vi "Command - On-Demand (SubVI) - B.vi"(0 "ESP Config":T2={"COM Port Input"="COM8", "Manual Command"={"Device Type"="", "Instance"="", "Command"="", "Sub-Command"="", "Parameters (Seperate by :)"=""}, "Device Type"="e", "Instance"="a", "Use Manual Command"=TRUE, "Timeout [msec]"=1000, "Read/Write Wait [msec]"=25}, 5 "ESP Table Cluster Ref":refnum<vi>, 7 "Display Cluster Ref":refnum<vi>) -> (4 "ESP Output":T3={"Write Command"="ea:DU:1", "Read String"="\u0006\u0001ea:00.000:00.000:00.036:00.004:AEA8\u0004", "Read Bytes"=12, "Bytes at Port"=12, "Response"="ea:00.000:00.000:00.036:00.004:AEA8", "ACK"=TRUE, "EOT"=TRUE, "NAK"=FALSE, "Parameters"=["00.000", "00.000", "00.036", "00.004"]}, 8 "On-Demand Header":string[](array[string]), 10 "On-Demand Data":string[](array[string]), 15 "ON Demand":errorcluster={"status"=FALSE, "code"=1073676294, "source"="VISA Read in ESP-D Read-Write (SubVI).vi->IO Board Evaluate.vi"})   [LabVIEW 2011]
panel:
  out "data 2":i32[](array[numeric])
  out "data":T1(array[cluster])
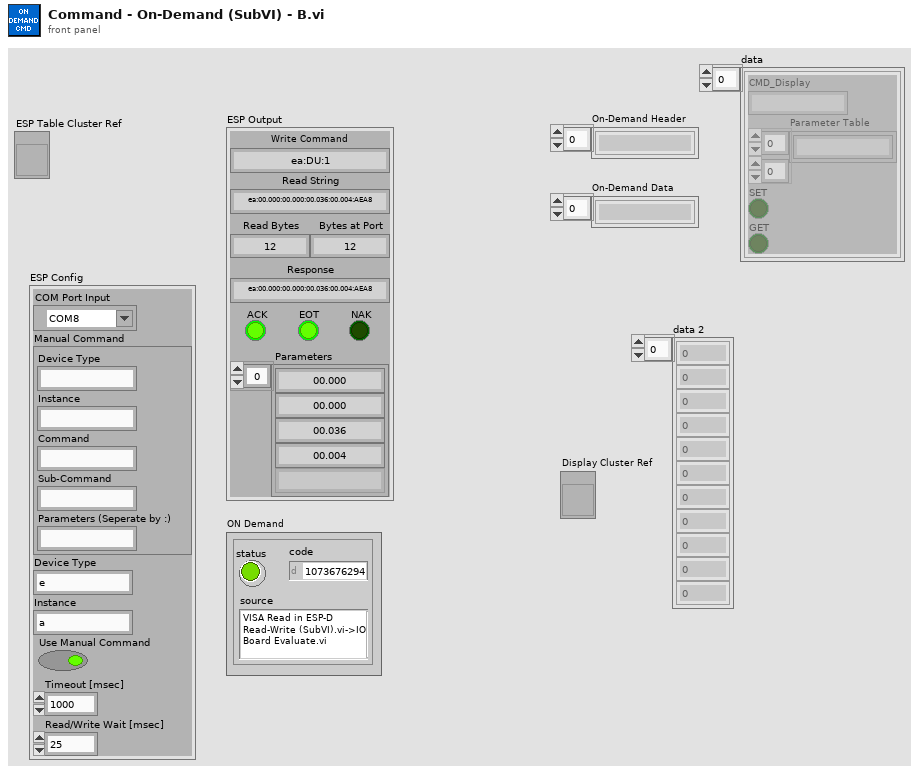
[diagram p1: front panel]
types:
  T1 = cluster{"CMD_Display":string, "Parameter Table":string[][], "SET":bool, "GET":bool}[]
  T2 = cluster{"COM Port Input":refnum<visa-resource-name>, "Manual Command":cluster{"Device Type":string, "Instance":string, "Command":string, "Sub-Command":string, "Parameters (Seperate by :)":string}, "Device Type":string, "Instance":string, "Use Manual Command":bool, "Timeout [msec]":u32, "Read/Write Wait [msec]":u32}
  T3 = cluster{"Write Command":string, "Read String":string, "Read Bytes":u32, "Bytes at Port":u32, "Response":string, "ACK":bool, "EOT":bool, "NAK":bool, "Parameters":string[]}
  T4 = cluster{"ON Demand Button":i32, "ON Demand Commands":i32, "Continuous Button":i32, "Continuous Commands":i32, "Error Button":i32, "Error Command":i32, "Status Button":i32, "Status Command":i32, "Digital Button":i32, "Digital Command":i32, "Save Table Button":i32, "Active Table":i32, "New Table Name":i32, "Table":i32}
  T5 = cluster{"Device Type":string, "Instance":string, "Command":string, "Sub-Command":string, "Parameters (Seperate by :)":string}
  T6 = cluster{"CMD_Display":string, "Parameter Table":string[][], "SET":bool, "GET":bool}
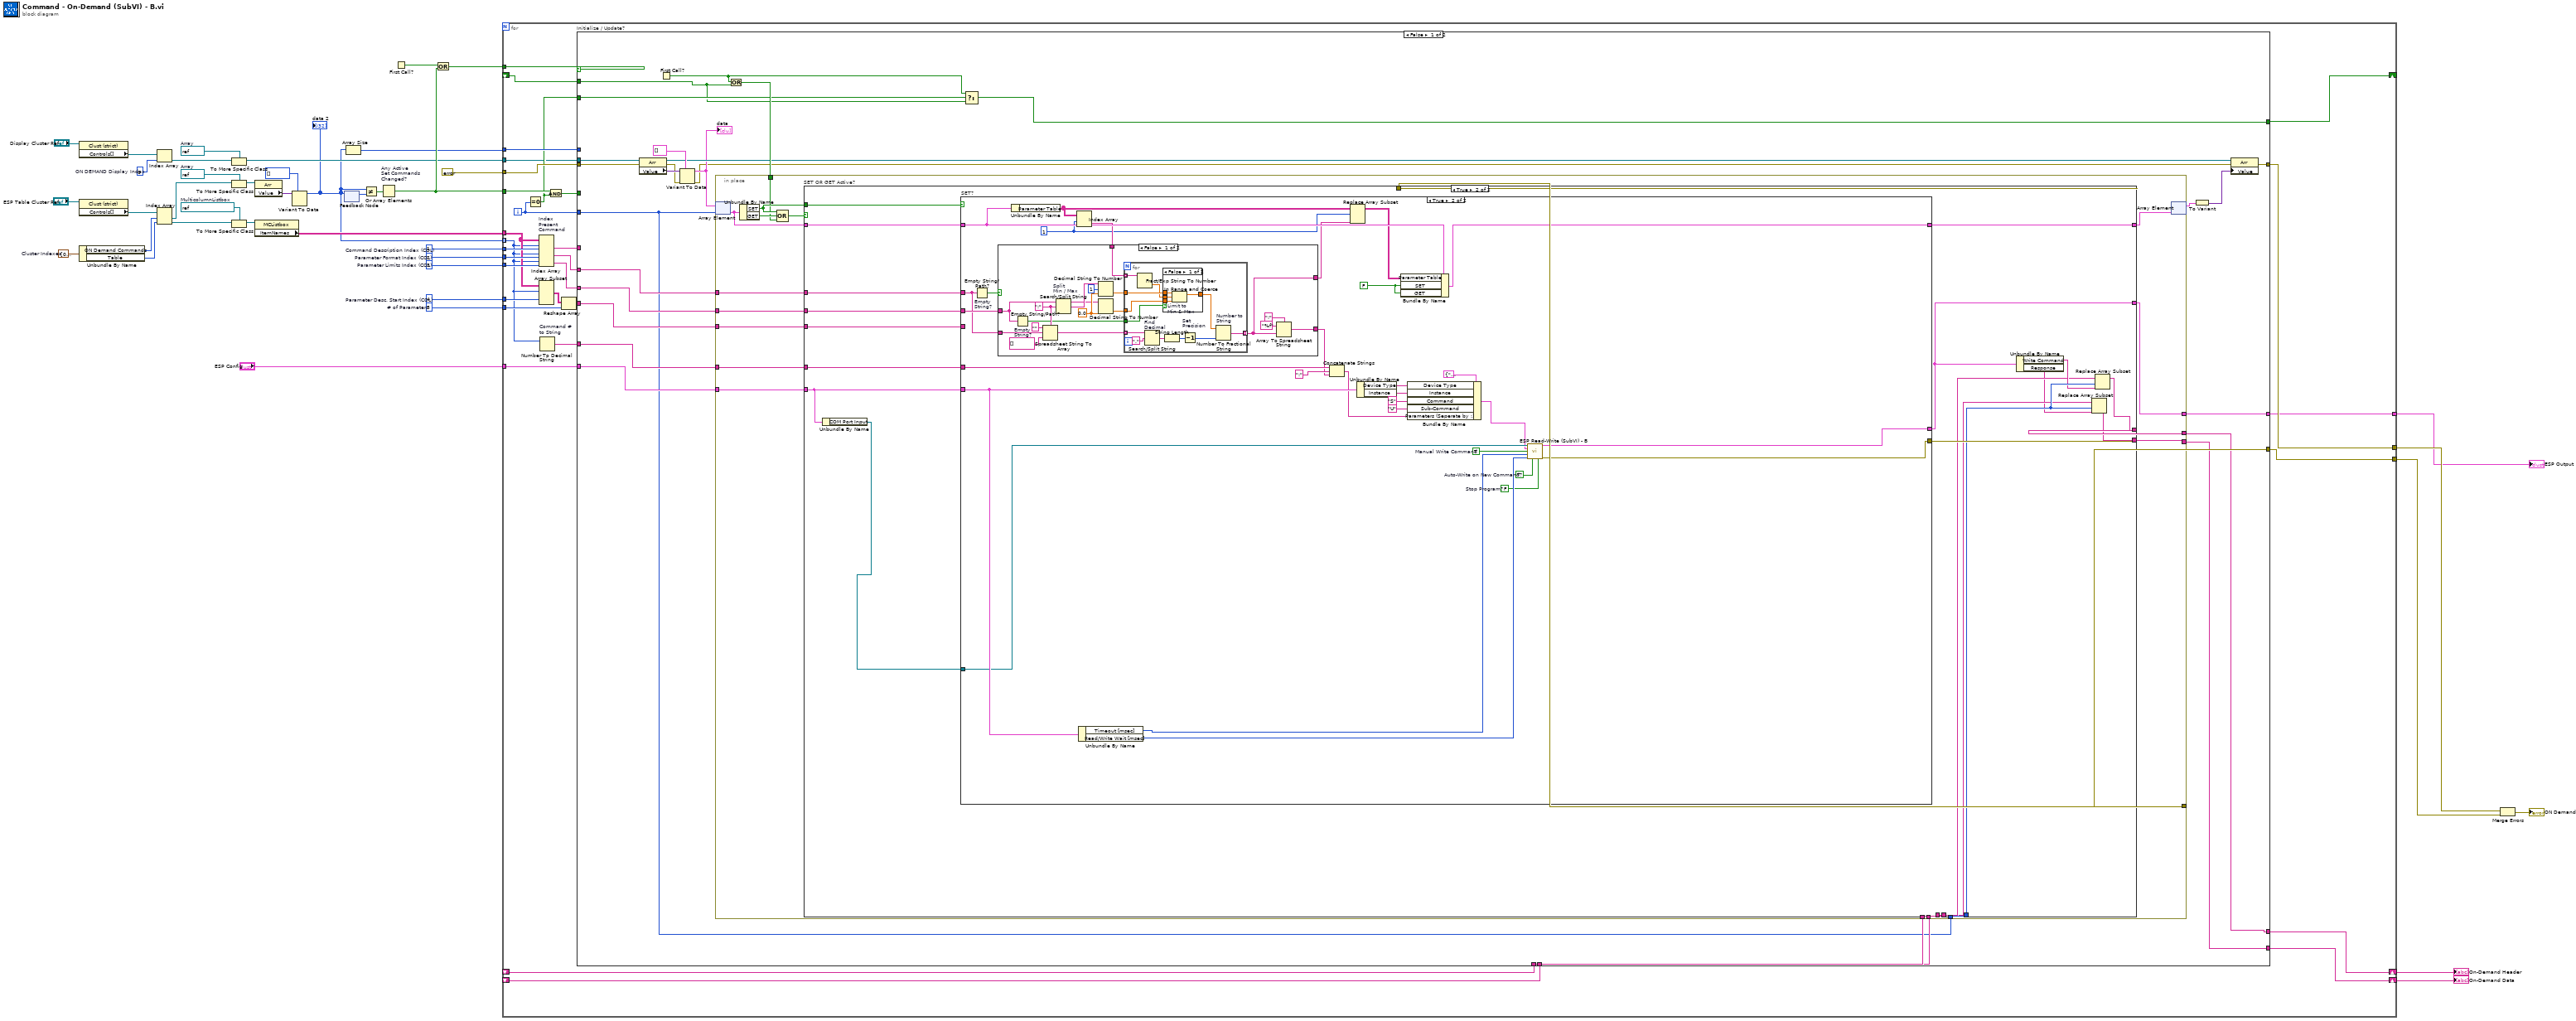
[diagram p0: block diagram]
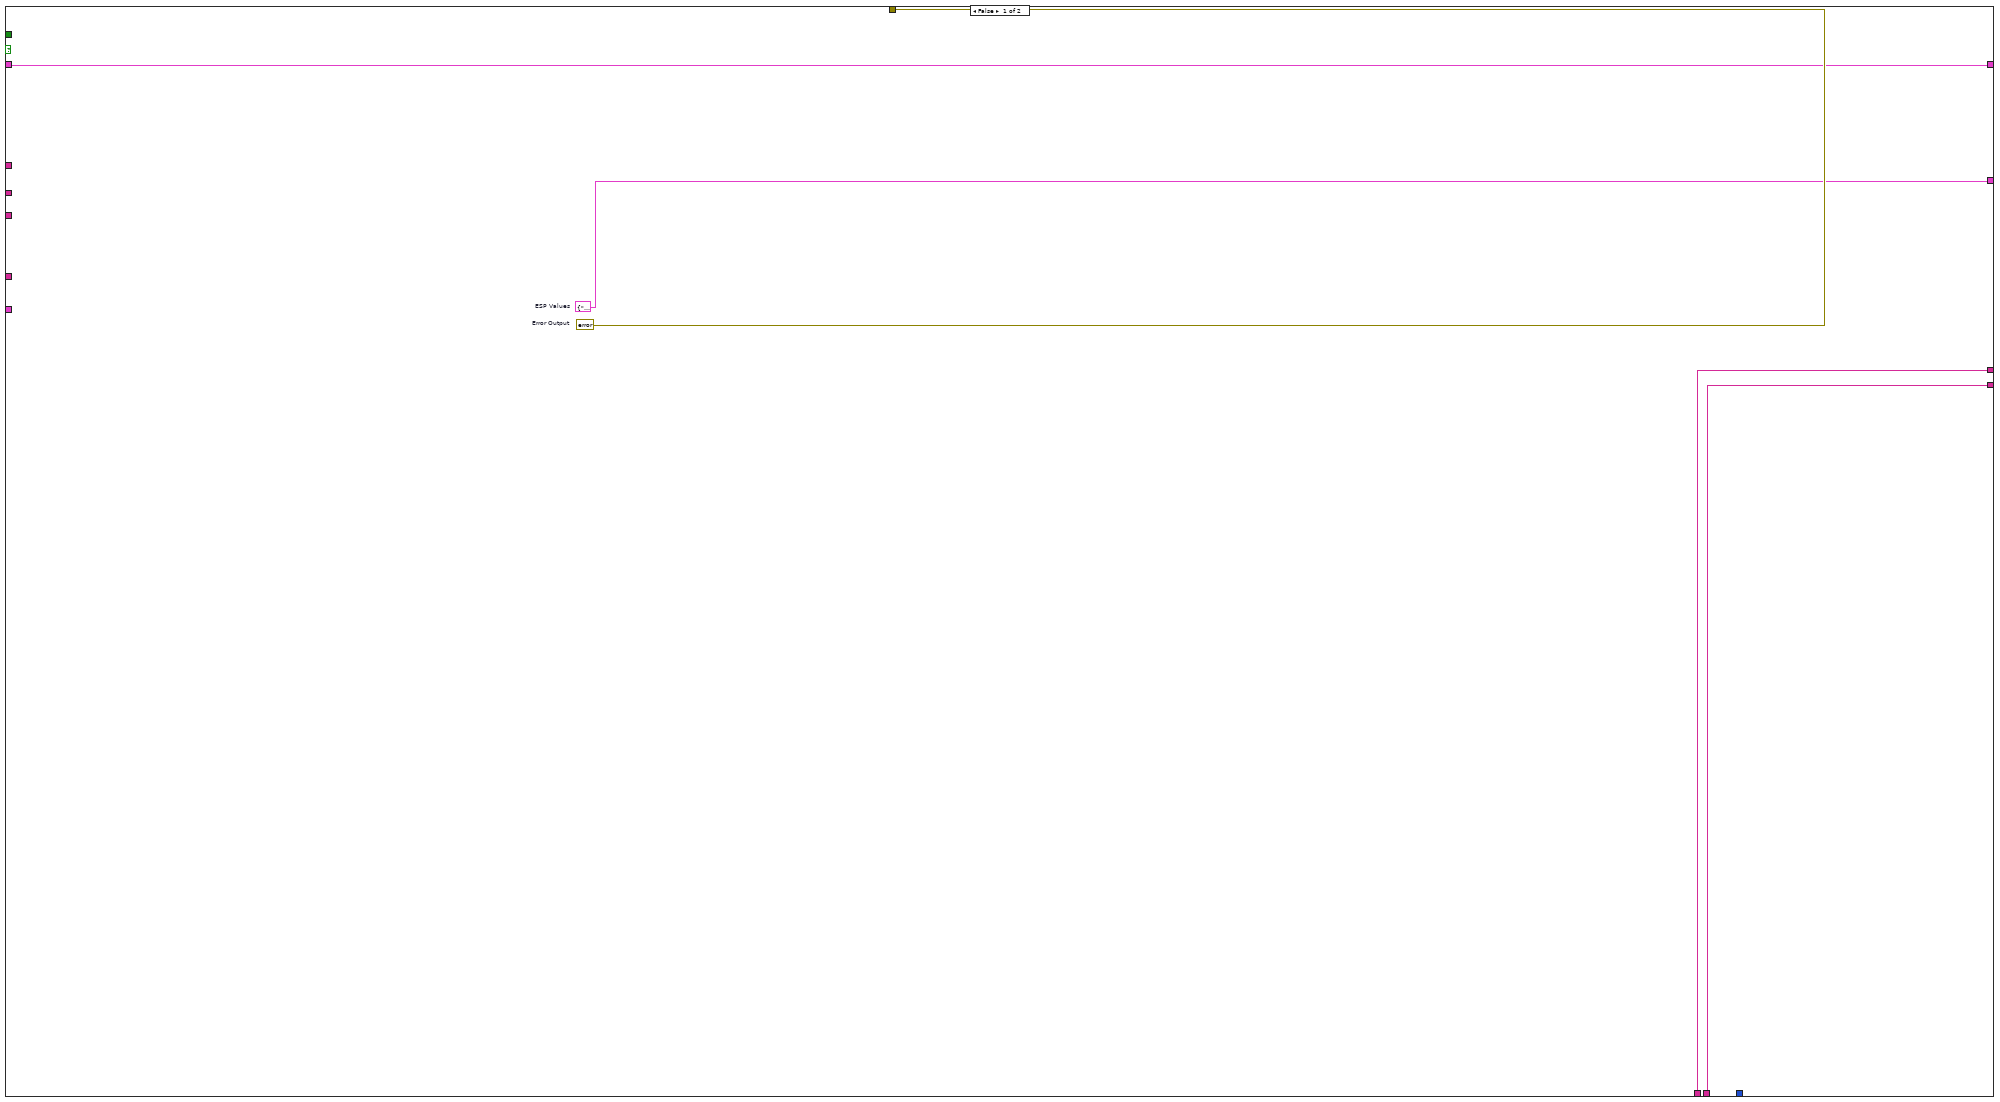
[diagram p2: hidden frame]
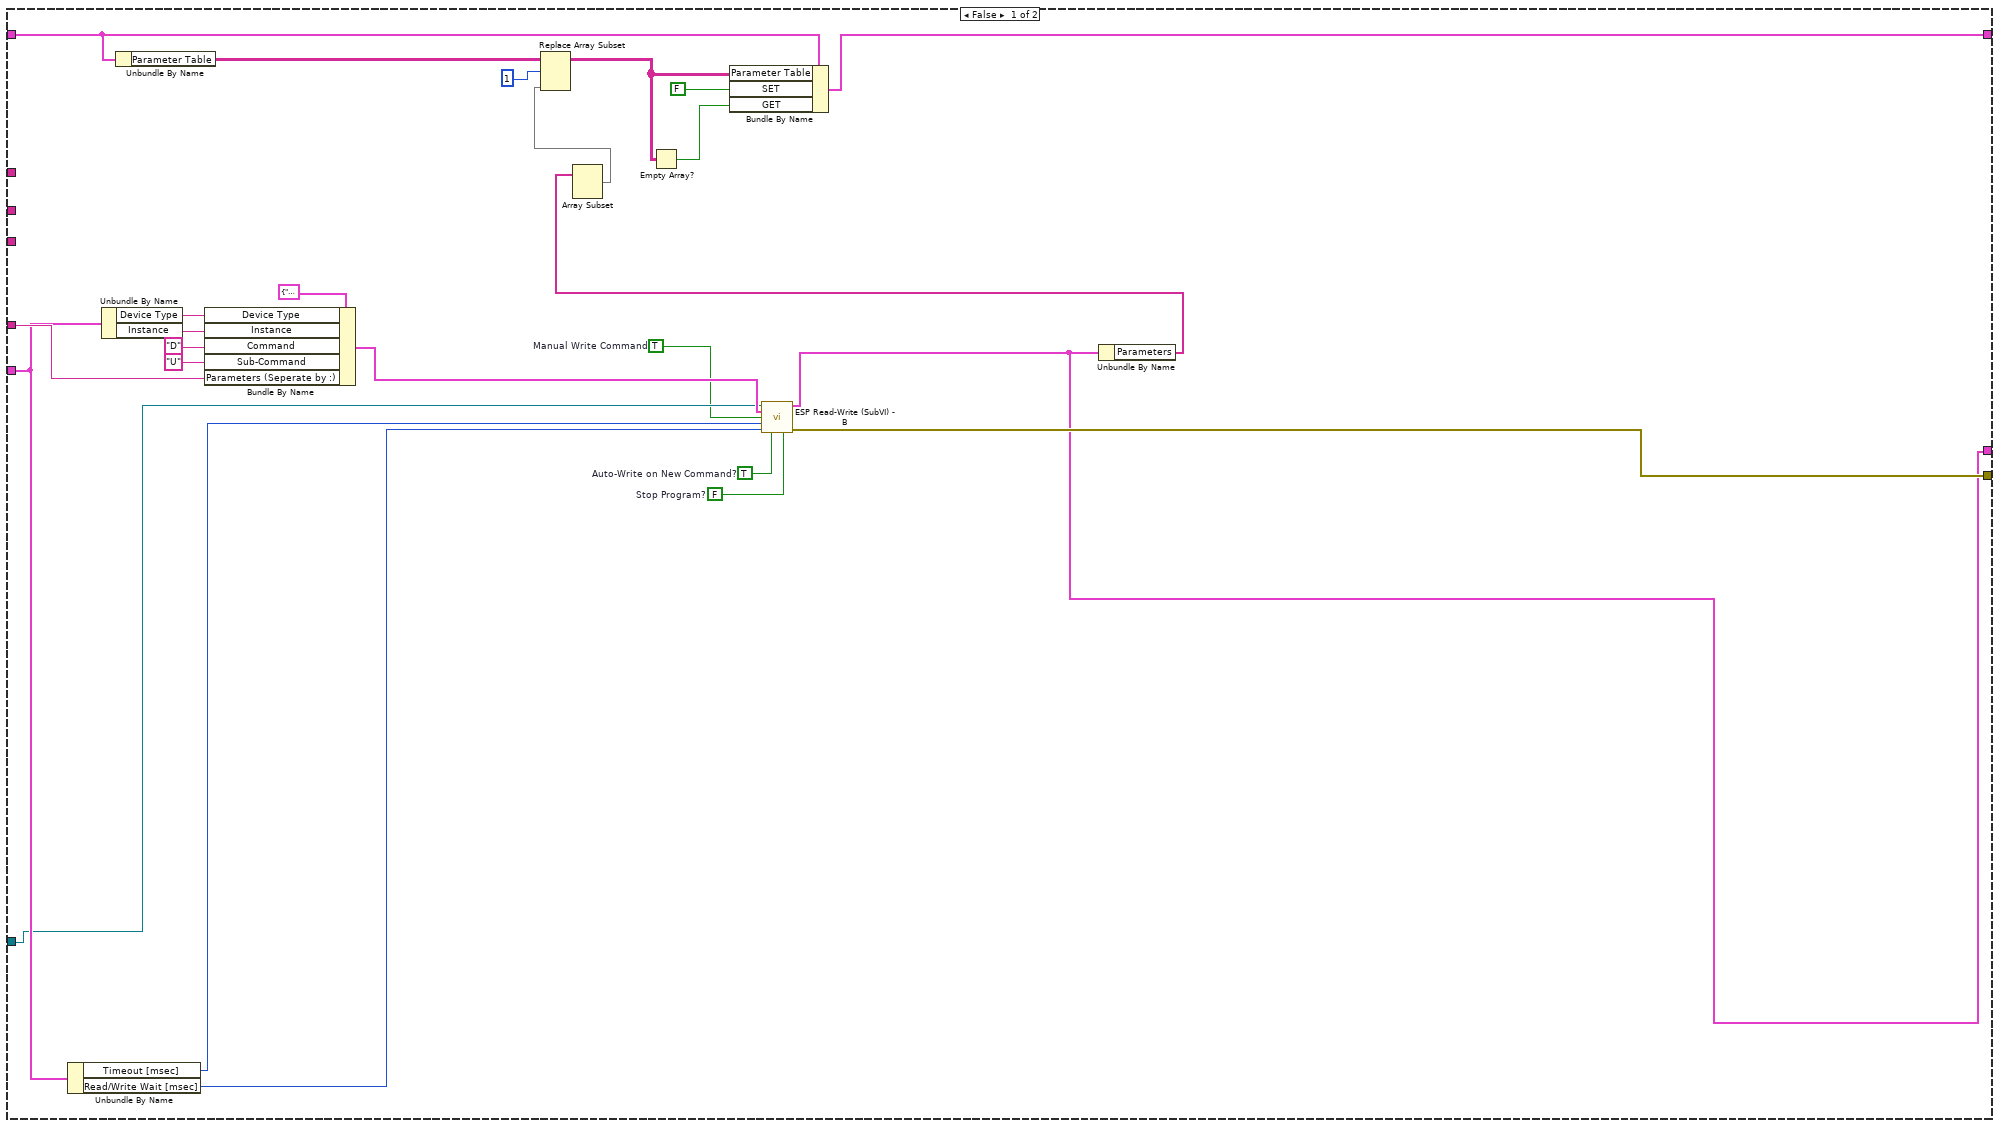
[diagram p3: hidden frame]
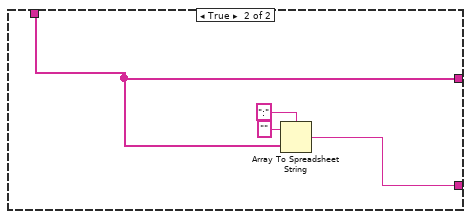
[diagram p5: hidden frame]
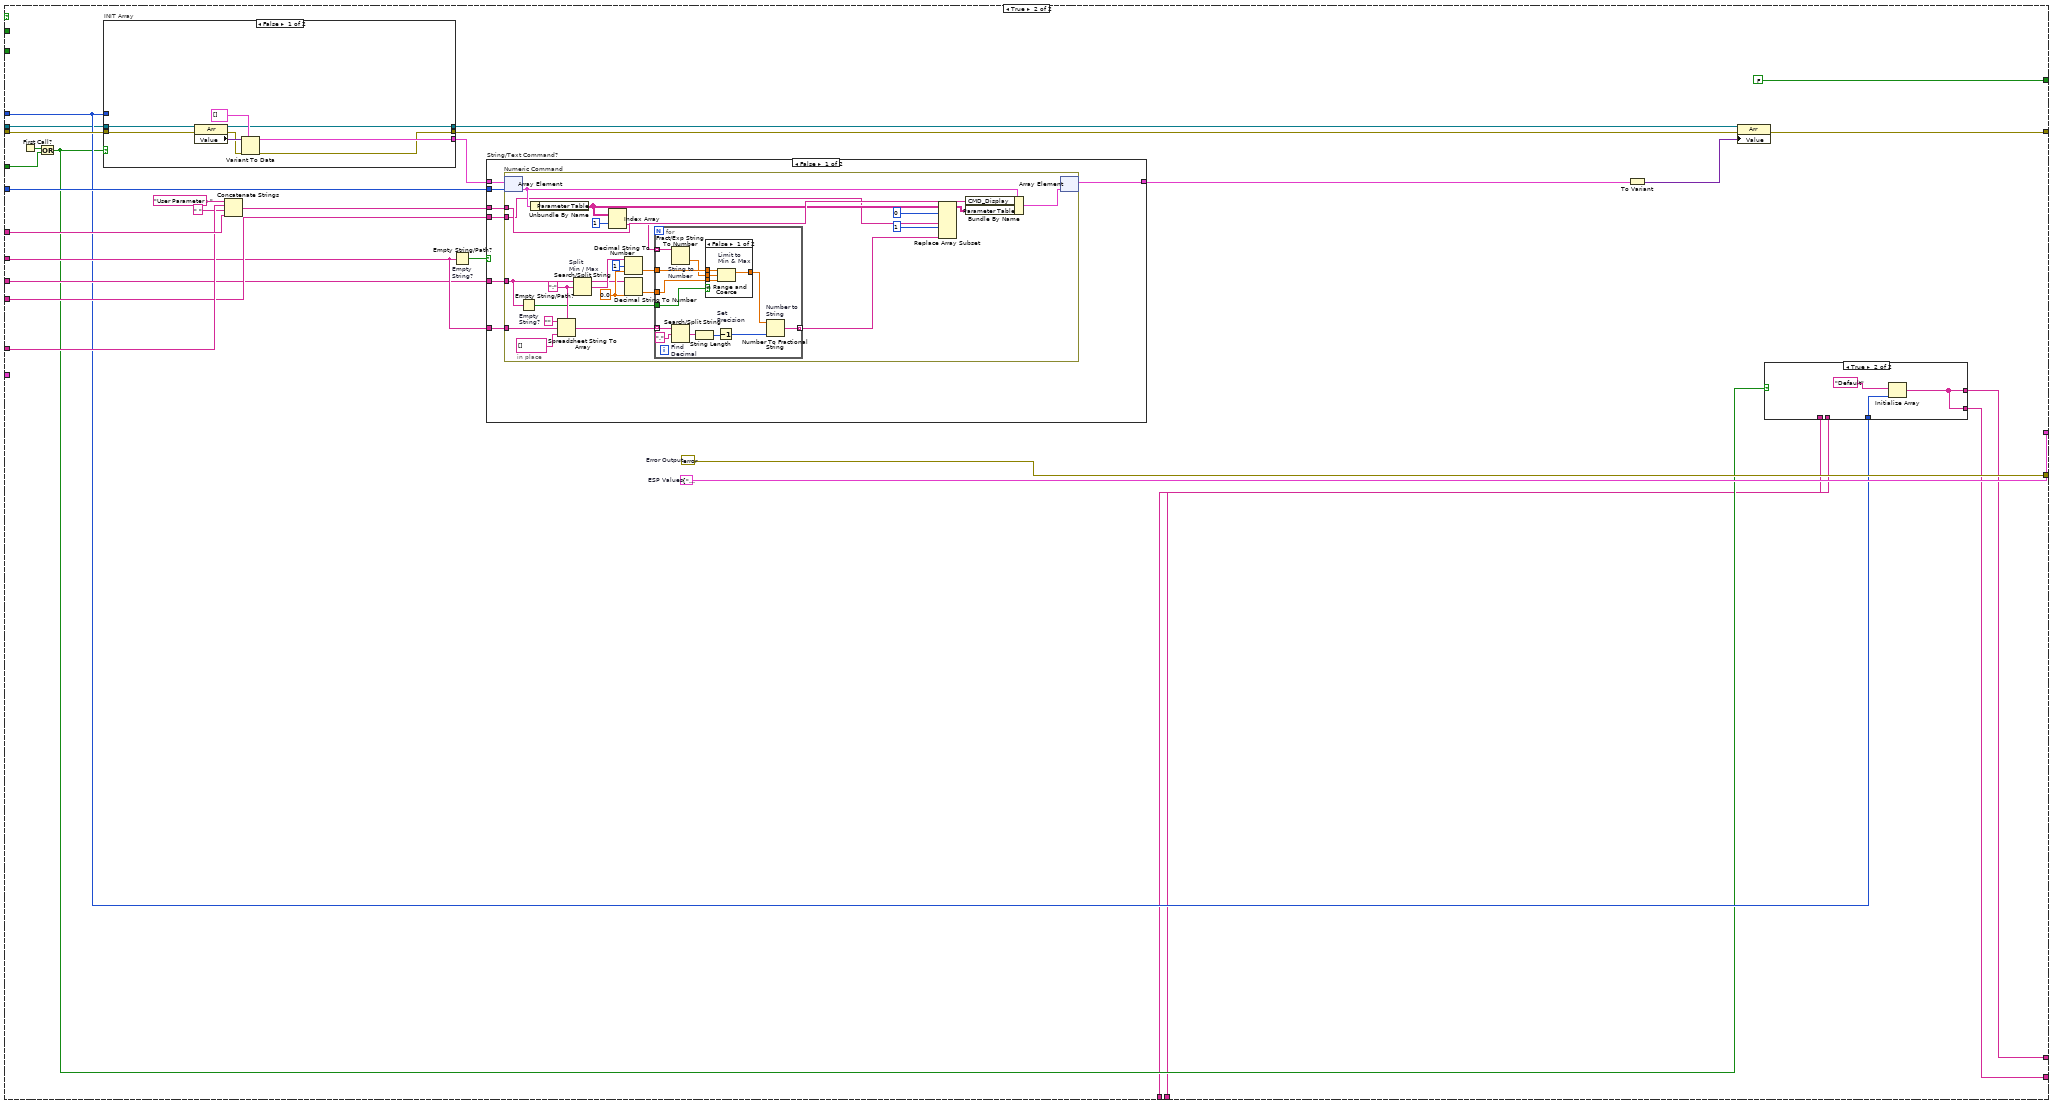
[diagram p6: hidden frame]
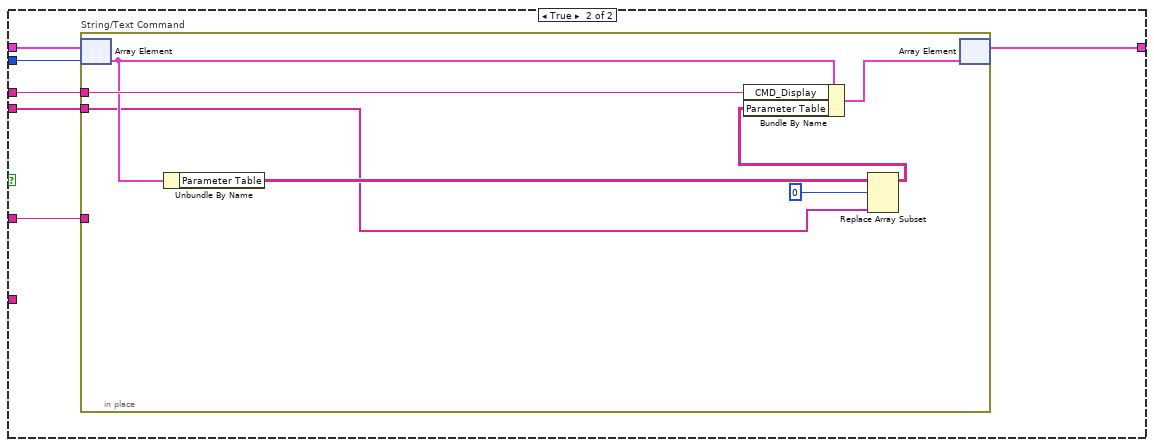
[diagram p9: hidden frame]
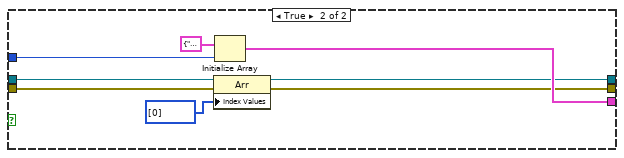
[diagram p10: hidden frame]
diagram:
  w2 = refnum<vi> refnum  # Array
  w4 = 0  # ON DEMAND Display Index
  w15 = T4 {"ON Demand Button"=0, "ON Demand Commands"=1, "Continuous Button"=2, "Continuous Commands"=3, "Error Button"=4, "Error Command"=5, "Status Button"=6, "Status Command"=7, "Digital Button"=8, "Digital Command"=9, "Save Table Button"=10, "Active Table"=11, "New Table Name"=12, "Table"=13}  # Cluster Indexes
  w18 = refnum<vi> refnum  # MulticolumnListbox
  w6 = refnum<vi> refnum  # Array
  w31 = 1  # Command Description Index (COL)
  w34 = 3  # # of Parameters
  w33 = 4  # Parameter Desc. Start Index (COL)
  w35 = 3  # Parameter Limits Index (COL)
  w36 = 2  # Parameter Format Index (COL)
  n1 = property class="Clust (strict)"(reference="Display Cluster Ref") -> ("Controls[]"=w5:refnum<vi>[])  [unwired: 1 in, 2 out]
  n2 = property class="Clust (strict)"(reference="ESP Table Cluster Ref") -> ("Controls[]"=w16:refnum<vi>[])  [unwired: 1 in, 2 out]
  n3 = Unbundle By Name(w15) -> ("ON Demand Commands"=w14:i32, "Table"=w13:i32)
  n4 = Index Array(array=w5, index=w4) -> (element=w3:refnum<vi>)
  n5 = Index Array(array=w16, index #1=w14, index #2=w13) -> (element #1=w10:refnum<vi>, element #2=w12:refnum<vi>)
  n6 = To More Specific Class(target class=w6, reference=w3) -> (specific class reference=w20:refnum<vi>)  [unwired: 1 in, 1 out]
  n7 = To More Specific Class(target class=w2, reference=w10) -> (specific class reference=w19:refnum<vi>)  [unwired: 1 in, 1 out]
  n8 = To More Specific Class(target class=w18, reference=w12) -> (specific class reference=w17:refnum<vi>)  [unwired: 1 in, 1 out]
  n9 = property class="Arr"(reference=w19) -> ("Value"=w8:variant)  [unwired: 1 in, 2 out]
  n10 = property class="MCListbox"(reference=w17) -> ("ItemNames"=w30:string[][])  [unwired: 1 in, 2 out]
  n11 = Variant To Data(type=i32[] [], Variant=w8) -> (data=w7:i32[])  [unwired: 1 in, 1 out]
  "data 2" <- w7
  n12 = feedback #1() -> (w27:i32[])  [unwired: 1 in]
  n13 = feedback-in #1(w7) -> ()
  n14 = Array Size(array=w7) -> (size(s)=w29:i32)
  n15 = Not Equal?(x=w7, y=w27) -> (x != y?=w28:bool[])
  n16 = Or Array Elements "Any Active\nSet Commands\nChanged?"(Boolean array=w28) -> (logical OR=w39:bool)
  n17 = First Call?() -> (First Call?: T/F=w38:bool)
  n18 = Or(x=w38, y=w39) -> (x .or. y?=w40:bool)
  n19 = for {
    tunnel: w36 -> [w70]
    tunnel: w35 -> [w69]
    tunnel: w34 -> [w68]
    tunnel: w33 -> [w67]
    tunnel: errorcluster {"status"=FALSE, "code"=0, "source"=""} -> [w66]
    tunnel: w31 -> [w65]
    tunnel: w7 -> [w53] mode=indexing
    tunnel: w30 -> [w60]
    tunnel: w29 -> [w59]
    tunnel: w39 -> [w56]
    tunnel: [w51] -> w26
    tunnel: [w55] -> w25
    tunnel: [w46] -> w24
    tunnel: "ESP Config" -> [w52]
    tunnel: w40 -> [w50]
    shift-right: [w49] -> _
    shift-left: _ -> [w48]
    shift-right: [w44] -> w22
    shift-left: _ -> [w45]
    shift-right: [w43] -> w21
    shift-left: _ -> [w42]
    tunnel: w20 -> [w41]
    i -> [w58]
    n20 = Equal To 0?(x=w58) -> (x = 0?=w47:bool)
    n21 = Index Array "Index\nPresent\nCommand"(array=w60, index (row) #1=w53, index (col) #1=w65, index (row) #2=w53, index (col) #2=w70, index (row) #3=w53, index (col) #3=w69) -> (element #1=w63:string, element #2=w62:string, element #3=w61:string)
    n22 = Array Subset(array=w60, index (row)=w53, index (col)=w67) -> (w71:string[][])  [unwired: 2 in]
    n23 = Number To Decimal String "Command #\nto String"(number=w53) -> (decimal integer string=w54:string)  [unwired: 1 in]
    n24 = And(x=w56, y=w47) -> (x .and. y?=w57:bool)
    n25 = Reshape Array(w71, w68) -> (w64:string[])
    n26 = case "Initialize / Update?" shown="False" w50 {
      tunnel: w63 -> [_ w263]
      tunnel: w66 -> [w77 w262]
      tunnel: w58 -> [w83 w260]
      tunnel: [w99 w261] -> w55
      tunnel: w54 -> [w95 w259]
      tunnel: w64 -> [w92 w258]
      tunnel: w62 -> [w97 w257]
      tunnel: w61 -> [w98 w256]
      tunnel: w59 -> [_ w242]
      tunnel: w57 -> [_ w255]
      tunnel: w52 -> [w96 _]
      tunnel: [w86 w246] -> w46
      tunnel: [w94 w245] -> w51
      tunnel: [w88 FALSE] -> w49
      tunnel: w48 -> [w87 _]
      tunnel: w47 -> [w90 _]
      tunnel: w45 -> [w85 w237]
      tunnel: [w82 w241] -> w44
      tunnel: [w81 w239] -> w43
      tunnel: w42 -> [w84 w238]
      tunnel: w41 -> [w78 w236]
      frame False {
        n27 = property class="Arr"(reference=w78, error in=w77) -> (reference out=w75:refnum<vi>, error out=w76:errorcluster, "Value"=w79:variant)
        n28 = First Call?() -> (First Call?: T/F=w89:bool)
        n29 = Variant To Data(error in=w76, type=T1 [], Variant=w79) -> (data=w74:T1, error out=w72:errorcluster)
        "data" <- w74
        n30 = Or(x=w89, y=w87) -> (x .or. y?=w91:bool)
        n31 = in-place {
          in-place-border: w98 -> [w117]
          in-place-border: w97 -> [w116]
          in-place-border: w96 -> [w114]
          in-place-border: w95 -> [w113]
          in-place-border: [w110] -> w86
          in-place-border: [w112] -> w94
          in-place-border: w92 -> [w111]
          in-place-border: w91 -> [w107]
          in-place-border: [w104] -> w82
          in-place-border: w85 -> [w103]
          in-place-border: [w102] -> w81
          in-place-border: w84 -> [w101]
          in-place-border: w83 -> [w100]
          n32 = in-place-array #2(w74, w83) -> (w115:T6)
          n33 = Unbundle By Name(w115) -> ("SET"=w109:bool, "GET"=w108:bool)
          n34 = Compound Arithmetic op=OR(w109, w108, w107) -> (w106:bool)
          n35 = case "SET OR GET Active?" shown="True" w106 {
            tunnel: w117 -> [_ w140]
            tunnel: w116 -> [_ w134]
            tunnel: w109 -> [_ w139]
            tunnel: w115 -> [w120 w136]
            tunnel: w114 -> [_ w124]
            tunnel: w113 -> [_ w138]
            tunnel: [w121 w132] -> w110
            tunnel: [w122 w137] -> w112
            tunnel: [w120 w135] -> w105
            tunnel: w111 -> [_ w133]
            tunnel: [w119 w129] -> w104
            tunnel: w103 -> [w119 w128]
            tunnel: [w118 w125] -> w102
            tunnel: w101 -> [w118 w127]
            tunnel: w100 -> [_ w131]
            frame False {
              w121 = T3 {"Write Command"="", "Read String"="", "Read Bytes"=0, "Bytes at Port"=0, "Response"="", "ACK"=FALSE, "EOT"=FALSE, "NAK"=FALSE, "Parameters"=[]}  # ESP Values
              w122 = errorcluster {"status"=FALSE, "code"=0, "source"=""}  # Error Output
            }
            frame True {
              n36 = Unbundle By Name(w124) -> ("COM Port Input"=w123:refnum<visa-resource-name>)
              n37 = case "SET?" shown="True" w139 {
                tunnel: w140 -> [_ w195]
                tunnel: w134 -> [_ w184]
                tunnel: w124 -> [w152 w190]
                tunnel: w138 -> [w164 w193]
                tunnel: [w147 w169] -> w132
                tunnel: [w148 w170] -> w137
                tunnel: w136 -> [w153 w180]
                tunnel: [w165 w181] -> w135
                tunnel: w133 -> [_ _]
                tunnel: w123 -> [w146 w174]
                frame False {
                  w142 = FALSE  # Stop Program?
                  w143 = TRUE  # Auto-Write on New Command?
                  w144 = TRUE  # Manual Write Command
                  n38 = Unbundle By Name(w152) -> ("Timeout [msec]"=w145:u32, "Read/Write Wait [msec]"=w141:u32)
                  n39 = Unbundle By Name(w152) -> ("Device Type"=w162:string, "Instance"=w161:string)
                  n40 = Unbundle By Name(w153) -> ("Parameter Table"=w156:string[][])
                  n41 = Bundle By Name(cluster=T5 {"Device Type"="", "Instance"="", "Command"="", "Sub-Command"="", "Parameters (Seperate by :)"=""}, "Device Type"=w162, "Instance"=w161, "Command"="D", "Sub-Command"="U", "Parameters (Seperate by :)"=w164) -> (w150:T5)
                  n42 = call "ESP Read-Write (SubVI) - B.vi"("COM Port Input"=w146, "Command Input"=w150, "Manual Write Command"=w144, "Timeout (ms)"=w145, "Write/Read Wait (ms)"=w141, "Auto-Write on New Command?"=w143, "Stop Program?"=w142) -> ("ESP Values"=w147:T3, "Error Output"=w148:errorcluster)  [unwired: 7 in]
                  n43 = Unbundle By Name(w147) -> ("Parameters"=w149:string[])
                  n44 = Array Subset(array=w149) -> (w155:string[])  [unwired: 2 in]
                  n45 = Replace Array Subset(array=w156, new element=w155, index (row)=1) -> (w154:string[][])  [unwired: 1 in]
                  n46 = Empty Array?(array=w154) -> (empty?=w151:bool)
                  n47 = Bundle By Name(cluster=w153, "Parameter Table"=w154, "SET"=FALSE, "GET"=w151) -> (w165:T6)
                }
                frame True {
                  w166 = FALSE  # Stop Program?
                  w171 = TRUE  # Auto-Write on New Command?
                  w172 = TRUE  # Manual Write Command
                  w177 = 1
                  w182 = FALSE
                  n48 = Empty String/Path? "Empty\nString?"(string/path=w184) -> (empty?=w183:bool)
                  n49 = Unbundle By Name(w180) -> ("Parameter Table"=w178:string[][])
                  n50 = Index Array(array=w178, index (row)=w177) -> (element=w179:string[])  [unwired: 1 in]
                  n51 = case shown="False" w183 {
                    tunnel: [w213 w234] -> w192
                    tunnel: w184 -> [w212 _]
                    tunnel: w195 -> [w211 _]
                    tunnel: [w197 w231] -> w175
                    tunnel: w179 -> [w196 w231]
                    frame False {
                      w203 = 0.0
                      w210 = ":" ("delimiter (Tab)")
                      n52 = Empty String/Path? "Empty\nString?"(string/path=w211) -> (empty?=w198:bool)
                      n53 = Spreadsheet String To Array(delimiter (Tab)=w210, format string="", spreadsheet string=w212, array type (2D Dbl)=string[] []) -> (array=w208:string[])
                      n54 = Search/Split String "Split\nMin / Max"(string=w211, search string/char (-)=w210) -> (substring before match=w202:string, match + rest of string=w204:string)  [unwired: 1 in, 1 out]
                      n55 = Decimal String To Number(string=w204, offset=1, default (0L)=w203) -> (number=w206:dbl)  [unwired: 1 out]
                      n56 = Decimal String To Number(string=w202, default (0L)=w203) -> (number=w207:dbl)  [unwired: 1 in, 1 out]
                      n57 = for {
                        tunnel: w208 -> [w221] mode=indexing
                        tunnel: w206 -> [w223]
                        tunnel: w207 -> [w224]
                        tunnel: [w217] -> w197 mode=indexing
                        tunnel: w196 -> [w215] mode=indexing
                        tunnel: w198 -> [w214]
                        n58 = Fract/Exp String To Number(string=w215) -> (number=w222:dbl)  [unwired: 3 in, 1 out]
                        n59 = Search/Split String "Find\nDecimal"(string=w221, search string/char (-)=".") -> (match + rest of string=w220:string)  [unwired: 1 in, 2 out]
                        n60 = case shown="False" w214 {
                          tunnel: w224 -> [w229 _]
                          tunnel: w223 -> [w228 _]
                          tunnel: w222 -> [w227 w230]
                          tunnel: [w226 w230] -> w216
                          frame False {
                            n61 = In Range and Coerce "Limit to\nMin & Max"(upper limit=w228, x=w227, lower limit=w229) -> (coerced(x)=w226:dbl)  [unwired: 1 out]
                          }
                          frame True {
                          }
                        }
                        n62 = String Length(string=w220) -> (length=w218:i32)
                        n63 = Decrement "Set\nPrecision"(x=w218) -> (x-1=w219:i32)
                        n64 = Number To Fractional String "Number to\nString"(number=w216, precision (6)=w219) -> (F-format string=w217:string)  [unwired: 2 in]
                      }
                      n65 = Array To Spreadsheet String(delimiter (Tab)=":", array=w197, 3:"%f" ("format string")) -> (spreadsheet string=w213:string)
                    }
                    frame True {
                      n66 = Array To Spreadsheet String(delimiter (Tab)=":", array=w231, 3:"" ("format string")) -> (spreadsheet string=w234:string)
                    }
                  }
                  n67 = Unbundle By Name(w190) -> ("Timeout [msec]"=w168:u32, "Read/Write Wait [msec]"=w167:u32)
                  n68 = Concatenate Strings(w193, ":" ("delimiter (Tab)"), w192) -> (w185:string)
                  n69 = Replace Array Subset(array=w178, new element=w175, index (row)=w177) -> (w176:string[][])  [unwired: 1 in]
                  n70 = Unbundle By Name(w190) -> ("Device Type"=w189:string, "Instance"=w188:string)
                  n71 = Bundle By Name(cluster=w180, "Parameter Table"=w176, "SET"=w182, "GET"=w182) -> (w181:T6)
                  n72 = Bundle By Name(cluster=T5 {"Device Type"="", "Instance"="", "Command"="", "Sub-Command"="", "Parameters (Seperate by :)"=""}, "Device Type"=w189, "Instance"=w188, "Command"="S", "Sub-Command"="U", "Parameters (Seperate by :)"=w185) -> (w173:T5)
                  n73 = call "ESP Read-Write (SubVI) - B.vi"("COM Port Input"=w174, "Command Input"=w173, "Manual Write Command"=w172, "Timeout (ms)"=w168, "Write/Read Wait (ms)"=w167, "Auto-Write on New Command?"=w171, "Stop Program?"=w166) -> ("ESP Values"=w169:T3, "Error Output"=w170:errorcluster)  [unwired: 7 in]
                }
              }
              n74 = Unbundle By Name(w132) -> ("Write Command"=w130:string, "Response"=w126:string)
              n75 = Replace Array Subset(array=w127, new element=w126, index=w131) -> (w125:string[])
              n76 = Replace Array Subset(array=w128, new element=w130, index=w131) -> (w129:string[])
            }
          }
          n77 = in-place-array #2(w105) -> (w93:T1)  [unwired: 1 out]
        }
        n78 = Select(t=w89, s=w90, f=w87) -> (s? t:f=w88:bool)
        n79 = To Variant(anything=w93) -> (Variant=w73:variant)
        n80 = property class="Arr"(reference=w75, error in=w72, "Value"=w73) -> (error out=w99:errorcluster)  [unwired: 1 out]
      }
      frame True {
        w246 = T3 {"Write Command"="", "Read String"="", "Read Bytes"=0, "Bytes at Port"=0, "Response"="", "ACK"=FALSE, "EOT"=FALSE, "NAK"=FALSE, "Parameters"=[]}  # ESP Values
        w245 = errorcluster {"status"=FALSE, "code"=0, "source"=""}  # Error Output
        n81 = First Call?() -> (First Call?: T/F=w247:bool)
        n82 = Or(x=w247, y=w255) -> (x .or. y?=w240:bool)
        n83 = case "INIT Array" shown="False" w240 {
          tunnel: [w332 w345] -> w253
          tunnel: w242 -> [_ w344]
          tunnel: w262 -> [w330 w341]
          tunnel: [w333 w342] -> w250
          tunnel: [w331 w340] -> w249
          tunnel: w236 -> [w334 w338]
          frame False {
            n84 = property class="Arr"(reference=w334, error in=w330) -> (reference out=w333:refnum<vi>, error out=w335:errorcluster, "Value"=w336:variant)
            n85 = Variant To Data(error in=w335, type=T1 [], Variant=w336) -> (data=w332:T1, error out=w331:errorcluster)
          }
          frame True {
            n86 = property class="Arr"(reference=w338, error in=w341, "Index Values"=u32[] [0]) -> (reference out=w342:refnum<vi>, error out=w340:errorcluster)
            n87 = Initialize Array(T6 {"CMD_Display"="", "Parameter Table"=[["", "", ""], ["", "", ""]], "SET"=FALSE, "GET"=FALSE} ("Read Cluster"), w344) -> (w345:T1)
          }
        }
        n88 = Concatenate Strings("User Parameter : " ("string"), w259, " ", w263) -> (w251:string)
        n89 = Empty String/Path? "Empty\nString?"(string/path=w257) -> (empty?=w248:bool)
        n90 = case "String/Text Command?" shown="False" w248 {
          tunnel: w257 -> [w275 _]
          tunnel: w256 -> [w274 w322]
          tunnel: w253 -> [w273 w321]
          tunnel: w260 -> [w272 w320]
          tunnel: w258 -> [w271 w319]
          tunnel: [w270 w318] -> w252
          tunnel: w251 -> [w269 w317]
          frame False {
            n91 = in-place "Numeric Command" {
              in-place-border: w275 -> [w289]
              in-place-border: w274 -> [w286]
              in-place-border: w269 -> [w288]
              in-place-border: w271 -> [w279]
              w293 = 0.0
              w299 = ":" ("delimiter (Tab)")
              n92 = in-place-array #3(w273, w272) -> (w283:T6)
              n93 = Empty String/Path? "Empty\nString?"(string/path=w286) -> (empty?=w285:bool)
              n94 = Unbundle By Name(w283) -> ("Parameter Table"=w284:string[][])
              n95 = Spreadsheet String To Array(delimiter (Tab)=w299, format string="", spreadsheet string=w289, array type (2D Dbl)=string[] []) -> (array=w298:string[])
              n96 = Search/Split String "Split\nMin / Max"(string=w286, search string/char (-)=w299) -> (substring before match=w292:string, match + rest of string=w294:string)  [unwired: 1 in, 1 out]
              n97 = Index Array(array=w284, index (row)=1) -> (element=w281:string[])  [unwired: 1 in]
              n98 = Decimal String To Number(string=w294, offset=1, default (0L)=w293) -> (number=w296:dbl)  [unwired: 1 out]
              n99 = Decimal String To Number(string=w292, default (0L)=w293) -> (number=w297:dbl)  [unwired: 1 in, 1 out]
              n100 = for {
                tunnel: w298 -> [w307] mode=indexing
                tunnel: w296 -> [w309]
                tunnel: w297 -> [w310]
                tunnel: [w303] -> w277 mode=indexing
                tunnel: w281 -> [w301] mode=indexing
                tunnel: w285 -> [w300]
                n101 = Fract/Exp String To Number "String to\nNumber"(string=w301) -> (number=w308:dbl)  [unwired: 3 in, 1 out]
                n102 = Search/Split String "Find\nDecimal"(string=w307, search string/char (-)=".") -> (match + rest of string=w306:string)  [unwired: 1 in, 2 out]
                n103 = String Length(string=w306) -> (length=w304:i32)
                n104 = case shown="False" w300 {
                  tunnel: w310 -> [w315 _]
                  tunnel: w309 -> [w314 _]
                  tunnel: w308 -> [w313 w316]
                  tunnel: [w312 w316] -> w302
                  frame False {
                    n105 = In Range and Coerce "Limit to\nMin & Max"(upper limit=w314, x=w313, lower limit=w315) -> (coerced(x)=w312:dbl)  [unwired: 1 out]
                  }
                  frame True {
                  }
                }
                n106 = Decrement "Set\nPrecision"(x=w304) -> (x-1=w305:i32)
                n107 = Number To Fractional String "Number to\nString"(number=w302, precision (6)=w305) -> (F-format string=w303:string)  [unwired: 2 in]
              }
              n108 = Replace Array Subset(array=w284, new element #1=w279, index (row) #1=0, new element #2=w277, index (row) #2=1) -> (w276:string[][])  [unwired: 2 in]
              n109 = Bundle By Name(cluster=w283, "CMD_Display"=w288, "Parameter Table"=w276) -> (w287:T6)
              n110 = in-place-array #3(w287) -> (w270:T1)  [unwired: 1 out]
            }
          }
          frame True {
            n111 = in-place "String/Text Command" {
              in-place-border: w322 -> [_]
              in-place-border: w317 -> [w329]
              in-place-border: w319 -> [w324]
              n112 = in-place-array #4(w321, w320) -> (w325:T6)
              n113 = Unbundle By Name(w325) -> ("Parameter Table"=w327:string[][])
              n114 = Replace Array Subset(array=w327, new element=w324, index (row)=0) -> (w323:string[][])  [unwired: 1 in]
              n115 = Bundle By Name(cluster=w325, "CMD_Display"=w329, "Parameter Table"=w323) -> (w328:T6)
              n116 = in-place-array #4(w328) -> (w318:T1)  [unwired: 1 out]
            }
          }
        }
        n117 = To Variant(anything=w252) -> (Variant=w235:variant)
        n118 = property class="Arr"(reference=w250, error in=w249, "Value"=w235) -> (error out=w261:errorcluster)  [unwired: 1 out]
        n119 = case shown="True" w240 {
          tunnel: w242 -> [_ w267]
          tunnel: [w265 w266] -> w241
          tunnel: [w264 w266] -> w239
          tunnel: w238 -> [w264 _]
          tunnel: w237 -> [w265 _]
          frame False {
          }
          frame True {
            n120 = Initialize Array("Default", w267) -> (w266:string[])
          }
        }
      }
    }
  }
  "ESP Output" <- w24
  "On-Demand Header" <- w22
  "On-Demand Data" <- w21
  n121 = Merge Errors(w25, w26) -> (→"ON Demand":errorcluster)
